vi "BasicScope_V1.vi"() -> ()   [LabVIEW 2011]
panel:
  out "strArrayOut":string[](array[string])
  out "大小":i32
  out "strArrayBuf":string[](array[string])
  out "mu32ArrayOut":u32[](array[numeric])
  in  "strArrayIn":string[](array[string])
  out "波形图表":dbl(graph)
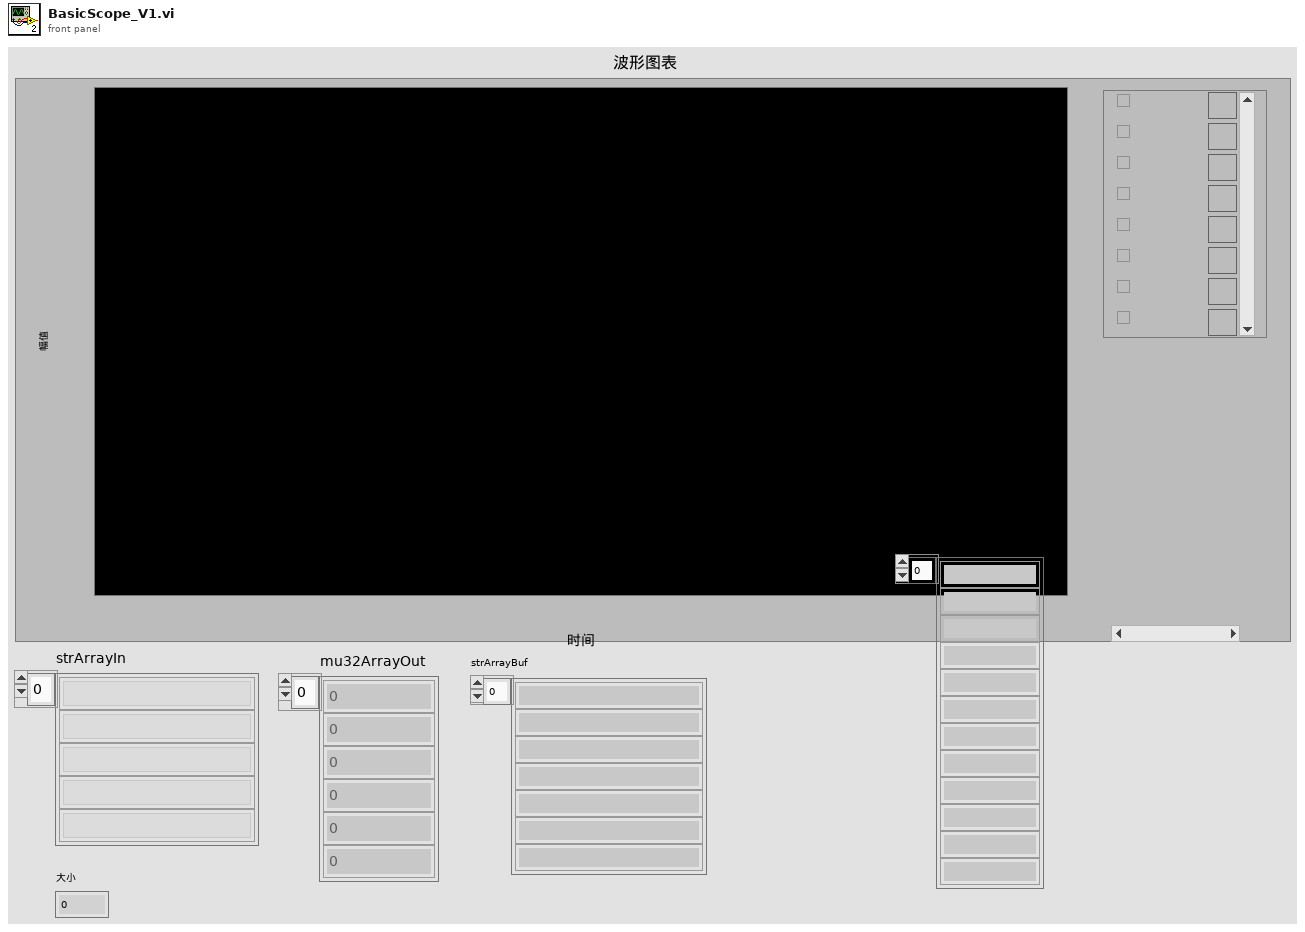
[diagram p1: front panel]
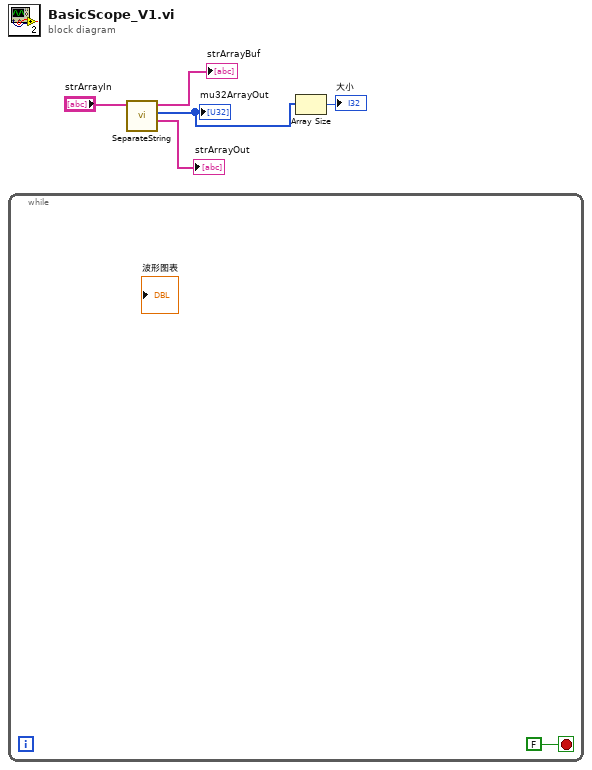
[diagram p0: block diagram]
diagram:
  n1 = while {
    stop <- FALSE stop-if-true
  }
  n2 = call "SeparateString.vi"("strArrayIn"="strArrayIn") -> ("strArrayOut"=→"strArrayOut":string[], "mu32ArrayOut"=w3:u32[], "strArrayBuf"=→"strArrayBuf":string[])  [unwired: 8 in]
  "mu32ArrayOut" <- w3
  n3 = Array Size(array=w3) -> (size(s)=→"大小":i32)
